vi "Spawn placeholder.vi"(11 "TEMPLATE Actor in":refnum<class "TEMPLATE Actor.lvclass">) -> (0 "Error out":errorcluster, 3 "TEMPLATE Actor out":refnum<class "TEMPLATE Actor.lvclass">)   [LabVIEW 2025, in "_Template.lvlib" / "Templates.lvlib" / "TEMPLATE Actor.lvlib" / "TEMPLATE Actor.lvclass"]
uses:
  TEMPLATE Actor.lvclass
  TEMPLATE Actor.lvclass/TEMPLATE Actor.ctl
  C:/git/jettl/src/jettl Tools/_Template/Templates/TEMPLATE Actor/TEMPLATE Actor/TEMPLATE Actor.lvclass
  C:/git/jettl/src/jettl/jettl/Actor/Actor.lvclass
  jettl/jettl/jettl.lvlib
  Static Child UIDs.ctl
  jettl/jettl/Transport/Queue/Queue.lvlib
  TEMPLATE Actor.lvlib
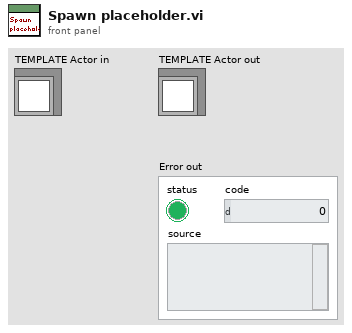
[diagram p1: front panel]
types:
  T1 = typedef "_Template.lvlib/Templates.lvlib/TEMPLATE Actor.lvlib/TEMPLATE Actor.lvclass/Static Child UIDs.ctl" = enum16{""}
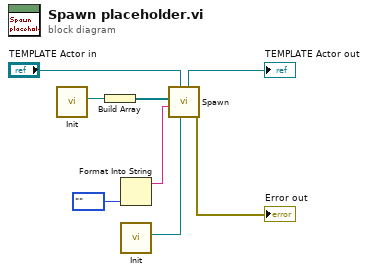
[diagram p0: block diagram]
diagram:
  n1 = call "Init.vi"() -> ("Actor"=w2:refnum<class "Actor.lvclass">)  [unwired: 11 in]
  n2 = Build Array(w2) -> (w1:refnum<class "Actor.lvclass">[])
  n3 = Format Into String(Static_Child_UIDs."" ("Static Child UIDs")) -> (resulting string=w5:string)  [unwired: 3 in, 1 out]
  n4 = call "Init.vi"() -> ("Transport"=w3:refnum<class "Transport.lvclass">)  [unwired: 11 in]
  n5 = call "Spawn.vi"("Transport"=w3, "Actor in"="TEMPLATE Actor in", "UID"=w5, "Actor Layers"=w1) -> ("Error out"=→"Error out":errorcluster, "Actor out"=→"TEMPLATE Actor out":refnum<class "TEMPLATE Actor.lvclass">)  [unwired: 6 in]
